vi "Begin.vi"(11 "Image Size":T1=enum."160x120") -> (0 "error out":errorcluster)   [LabVIEW 2012]
doc: "Called before other user functions, this VI is expected to open initial I/O refnums, load in file data, and do all program initialization. Notice that the <B>error out</B> terminal is simply used for data flow. Wiring it to other structures or subVIs ensures that this VI runs first."
uses:
  <vilib>/Rock Robotics/WPI/Camera/WPI_CameraImageSize.ctl
  <vilib>/Rock Robotics/WPI/Camera/WPI_CameraWhite Balance Values.ctl
  <vilib>/Rock Robotics/WPI/Camera/WPI_CameraExposure Values.ctl
  <vilib>/Rock Robotics/WPI/Camera/WPI_CameraFrameRate.ctl
  <vilib>/Rock Robotics/WPI/DriverStation/WPI_DriverStationRobotMode2.ctl
  <vilib>/Rock Robotics/WPI/Joystick/WPI_JoystickDeviceEnum.ctl
  <vilib>/Rock Robotics/SystemInterfaces/DIO/FPGA_DIOPWMChannel.ctl
  <vilib>/Rock Robotics/WPI/SafetyOutput/WPI_SafetyOutputConfigMenu.ctl
  <vilib>/Rock Robotics/SystemInterfaces/DIO/FPGA_DIORelayChannel.ctl
  <vilib>/Rock Robotics/SystemInterfaces/DIO/FPGA_DIOChannel.ctl
  <vilib>/Rock Robotics/WPI/Solenoid/WPI_SolenoidChannel.ctl
  <vilib>/Rock Robotics/SystemInterfaces/Typedef/FPGA_TypedefDigitalModule.ctl
  Robot Global Data.vi
  <vilib>/Rock Robotics/WPI/RobotDrive/WPI_RobotDriveOpen4MotorWithJaguar.vi
  <vilib>/Rock Robotics/WPI/MotorControl/WPI_MotorControlOpen Victor.vi
  <vilib>/Rock Robotics/WPI/Solenoid/WPI_SolenoidOpenSingle.vi
  <vilib>/Rock Robotics/WPI/Compressor/WPI_CompressorGetSetRefNum.vi
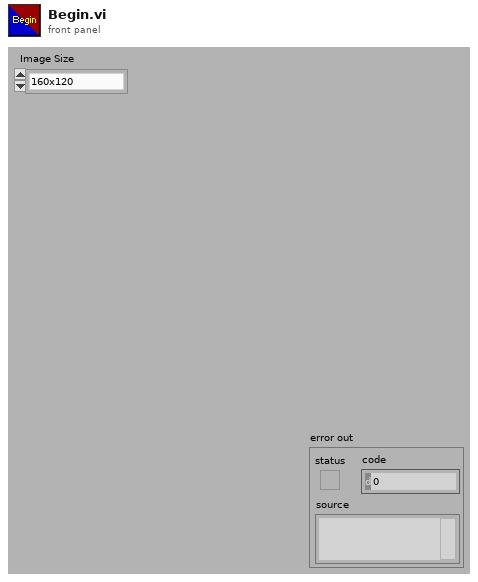
[diagram p1: front panel]
types:
  T1 = typedef "WPI_CameraImageSize.ctl" = enum16{"640x480", "320x240", "160x120"}
  T2 = typedef "FPGA_DIOPWMChannel.ctl" = enum8{"PWM 1", "PWM 2", "PWM 3", "PWM 4", "PWM 5", "PWM 6", "PWM 7", "PWM 8", "PWM 9", "PWM 10", "Invalid"}
  T3 = typedef "WPI_JoystickDeviceEnum.ctl" = enum16{"USB 1", "USB 2", "USB 3", "USB 4", "Kinect 1", "Kinect 2"}
  T4 = typedef "WPI_SafetyOutputConfigMenu.ctl" = enum16{"Enable", "Disable"}
  T5 = typedef "WPI_DriverStationRobotMode2.ctl" = enum16{"Autonomous Disabled", "Autonomous Enabled", "Teleop Disabled", "Teleop Enabled", "Timeout", "Finish", "Test Disabled", "Test Enabled"}
  T6 = typedef "WPI_CameraFrameRate.ctl" = u32
  T7 = typedef "WPI_CameraExposure Values.ctl" = enum16{"Auto", "Flicker-free 50 Hz", "Flicker-free 60 Hz", "Hold current"}
  T8 = typedef "WPI_CameraWhite Balance Values.ctl" = enum16{"Auto", "Fixed indoor", "Fixed outdoor 1", "Fixed outdoor 2", "Fixed fluorescent 1", "Fixed fluorescent 2", "Hold current"}
  T9 = typedef "WPI_SolenoidChannel.ctl" = enum8{"Solenoid 1", "Solenoid 2", "Solenoid 3", "Solenoid 4", "Solenoid 5", "Solenoid 6", "Solenoid 7", "Solenoid 8", "Invalid"}
  T10 = typedef "FPGA_DIOChannel.ctl" = enum8{"DIO 1", "DIO 2", "DIO 3", "DIO 4", "DIO 5", "DIO 6", "DIO 7", "DIO 8", "DIO 9", "DIO 10", "DIO 11", "DIO 12", "DIO 13", "DIO 14", "Invalid"}
  T11 = typedef "FPGA_DIORelayChannel.ctl" = enum8{"Relay 1", "Relay 2", "Relay 3", "Relay 4", "Relay 5", "Relay 6", "Relay 7", "Relay 8", "Invalid"}
  T12 = typedef "FPGA_TypedefDigitalModule.ctl" = enum16{"Digital Module 1", "Digital Module 2"}
  T13 = typedef "WPI_SolenoidDevRef.ctl" = cluster{"DevStatus":errorcluster, "Solenoid Module":T14, "Forward Solenoid Channel":T9, "Reverse Solenoid Channel":T9}
  T14 = typedef "FPGA_TypedefSolenoidModule.ctl" = enum16{"Solenoid Module 1", "Solenoid Module 2"}
  T15 = typedef "WPI_CompressorDevRef.ctl" = cluster{"DevStatus":errorcluster, "DigitalInputDevRef":T16, "RelayDevRef":T17}
  T16 = typedef "WPI_DigitalInputDevRef.ctl" = cluster{"DevStatus":errorcluster, "DIO Channel":T10, "Digital Module":T12}
  T17 = typedef "WPI_RelayDevRef.ctl" = cluster{"DevStatus":errorcluster, "Relay Channel":T11, "Digital Module":T12, "Relay Direction":T18}
  T18 = typedef "WPI_RelayDirection.ctl" = enum16{"Both directions", "Forward only", "Reverse only"}
  T19 = typedef "FPGA_WatchdogDevRef.ctl" = cluster{"DevStatus":errorcluster}
  T20 = typedef "WPI_RobotDriveDevRef.ctl" = cluster{"DevStatus":errorcluster, "Motors[]":T21[], "Square Inputs":bool, "Max Output":dbl, "Isochronous":bool}
  T21 = typedef "WPI_MotorControlDeviceRef.ctl" = cluster{"DeviceStatus":errorcluster, "Type":enum16{"PWM", "CAN"}, "PWM":cluster{"Digital Module":T12, "PWM Channel":T2, "DeadBand":T22}, "CAN":cluster{"Device Number":u8, "Control Mode":T23, "Semaphore":T24, "Max Vout":dbl}, "Invert":bool, "TransformRef":T25, "InvTransformRef":T25}
  T22 = typedef "WPI_PWMDeadband.ctl" = cluster{"Name":string, "maxPositivePwm":i32, "minPositivePwm":i32, "centerPwm":i32, "maxNegativePwm":i32, "minNegativePwm":i32, "angularRange":u16}
  T23 = typedef "WPI_CANJaguar_ControlMode.ctl" = enum8{"Percent VBus", "Current", "Speed", "Position", "Voltage"}
  T24 = typedef "Semaphore RefNum" = refnum<k1>
  T25 = typedef "WPI_PWMTransform_ConPane.ctl" = refnum<vi>
  T26 = typedef "WPI_JoystickDevRef.ctl" = cluster{"Device":T3}
  T27 = typedef "WPI_CameraDevRef.ctl" = cluster{"Camera Address":string, "CameraStatus":errorcluster, "Acquire Image Notifier":refnum<notifier>}
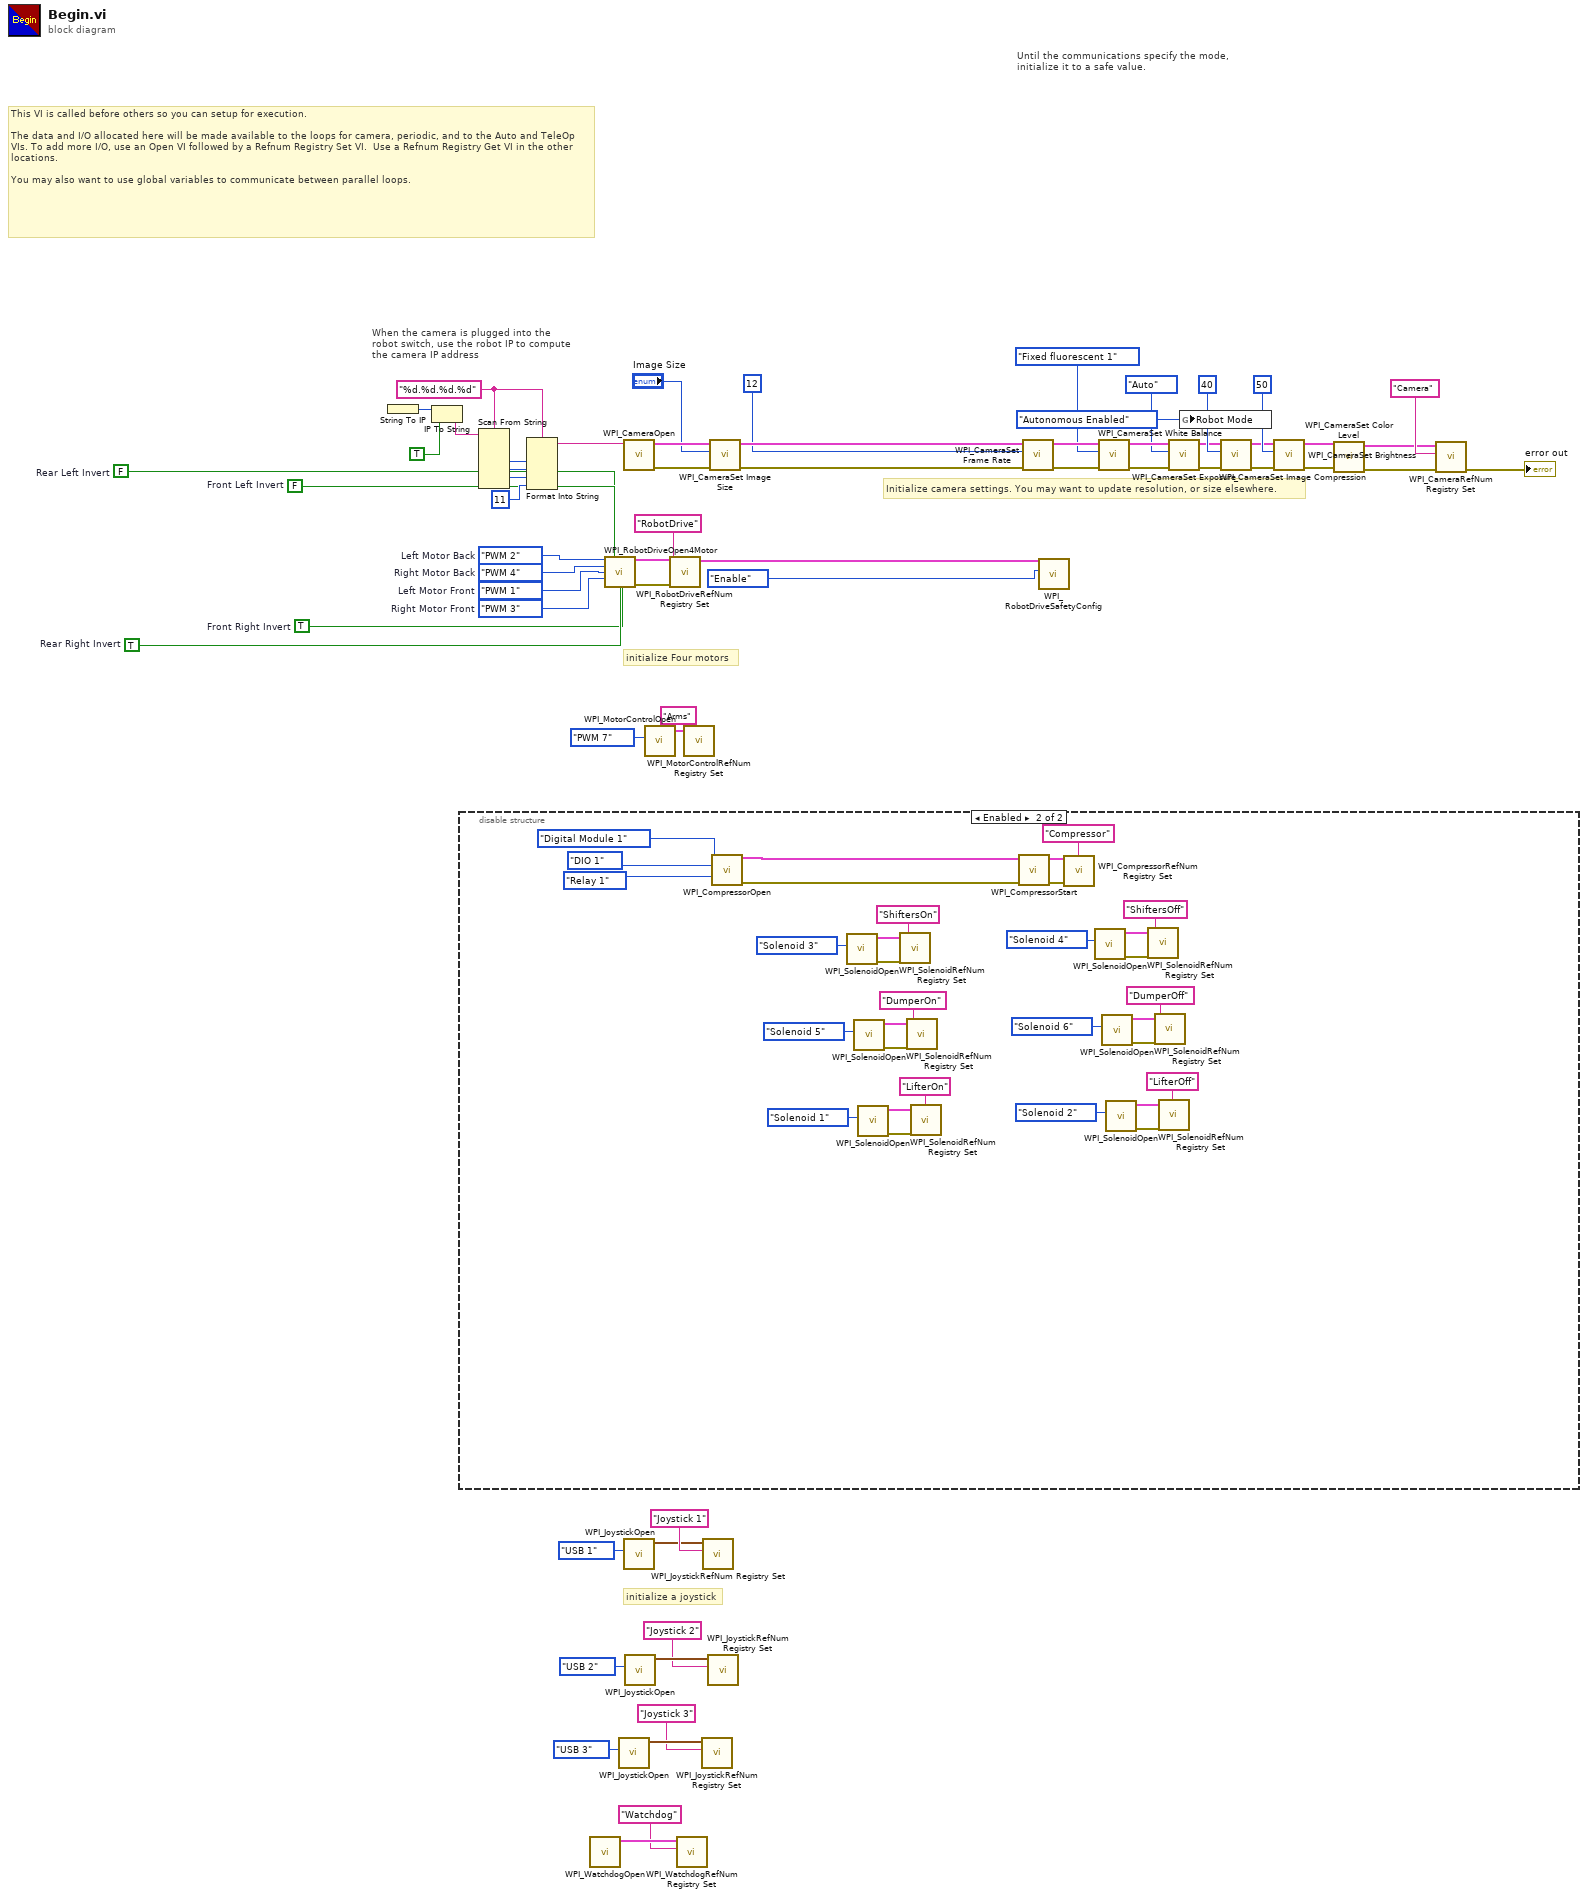
[diagram p0: block diagram]
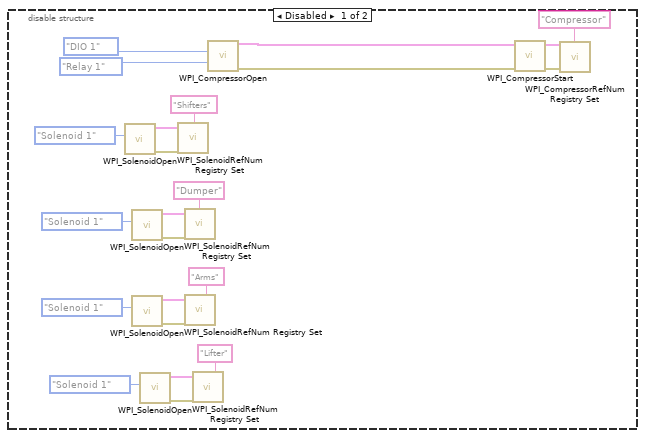
[diagram p2: hidden frame]
diagram:
  w16 = TRUE  # Front Right Invert
  w17 = FALSE  # Front Left Invert
  w22 = FPGA_DIOPWMChannel."PWM 4"  # Right Motor Back
  w19 = FPGA_DIOPWMChannel."PWM 3"  # Right Motor Front
  w21 = FPGA_DIOPWMChannel."PWM 2"  # Left Motor Back
  w20 = FPGA_DIOPWMChannel."PWM 1"  # Left Motor Front
  w15 = FALSE  # Rear Left Invert
  w18 = TRUE  # Rear Right Invert
  w35 = "%d.%d.%d.%d" ("format string")
  # "This VI is called before others so you can setup for execution.\n\nThe data and I/O allocated here will be made available to the loops for camera, periodic, and to the Auto and TeleOp VIs. To add more I/O, use an Open VI followed by a Refnum Registry Set VI.  Use a Refnum Registry Get VI in the other locations.\n\nYou may also want to use global variables to communicate between parallel loops."
  # "initialize a joystick"
  # "Until the communications specify the mode,\ninitialize it to a safe value."
  # "When the camera is plugged into the\nrobot switch, use the robot IP to compute\nthe camera IP address"
  # "initialize Four motors"
  # "Initialize camera settings. You may want to update resolution, or size elsewhere."
  n1 = String To IP() -> (0:w42:u32)  [unwired: 1 in]
  n2 = IP To String(1:TRUE ("dot notation? (F)"), 2:w42) -> (0:w40:string)
  n3 = disable-structure shown="Enabled" {
    frame Disabled {
      n4 = call-poly <vilib>:"WPI_SolenoidOpen.vi"("Solenoid Channel"=WPI_SolenoidChannel."Solenoid 1") -> ("error out"=w75:errorcluster, "SolenoidDevRef"=w76:T13)  [unwired: 9 in]
      n5 = call-poly <vilib>:"WPI_SolenoidOpen.vi"("Solenoid Channel"=WPI_SolenoidChannel."Solenoid 1") -> ("error out"=w71:errorcluster, "SolenoidDevRef"=w72:T13)  [unwired: 9 in]
      n6 = call-poly <vilib>:"WPI_SolenoidOpen.vi"("Solenoid Channel"=WPI_SolenoidChannel."Solenoid 1") -> ("error out"=w67:errorcluster, "SolenoidDevRef"=w68:T13)  [unwired: 9 in]
      n7 = call-poly <vilib>:"WPI_SolenoidOpen.vi"("Solenoid Channel"=WPI_SolenoidChannel."Solenoid 1") -> ("error out"=w63:errorcluster, "SolenoidDevRef"=w64:T13)  [unwired: 9 in]
      n8 = call <vilib>:"WPI_SolenoidRefNum Registry Set.vi"("error in (no error)"=w75, "refnum name"="Shifters", "SolenoidDevRef"=w76) -> ()  [unwired: 7 in, 2 out]
      n9 = call <vilib>:"WPI_SolenoidRefNum Registry Set.vi"("error in (no error)"=w71, "refnum name"="Dumper", "SolenoidDevRef"=w72) -> ()  [unwired: 7 in, 2 out]
      n10 = call <vilib>:"WPI_SolenoidRefNum Registry Set.vi"("error in (no error)"=w67, "refnum name"="Arms", "SolenoidDevRef"=w68) -> ()  [unwired: 7 in, 2 out]
      n11 = call <vilib>:"WPI_SolenoidRefNum Registry Set.vi"("error in (no error)"=w63, "refnum name"="Lifter", "SolenoidDevRef"=w64) -> ()  [unwired: 7 in, 2 out]
      n12 = call <vilib>:"WPI_CompressorOpen.vi"("Pressure Switch DIO Channel"=FPGA_DIOChannel."DIO 1", "Relay Channel"=FPGA_DIORelayChannel."Relay 1") -> ("CompressorDevRef"=w81:T15, "error out"=w82:errorcluster)  [unwired: 12 in]
      n13 = call <vilib>:"WPI_CompressorStart.vi"("error in (no error)"=w82, "CompressorDevRef"=w81) -> ("error out"=w79:errorcluster, "CompressorDevRef"=w80:T15)  [unwired: 8 in]
      n14 = call <vilib>:"WPI_CompressorRefNum Registry Set.vi"("error in (no error)"=w79, "refnum name"="Compressor", "CompressorDevRef"=w80) -> ()  [unwired: 7 in, 2 out]
    }
    frame Enabled {
      n15 = call <vilib>:"WPI_CompressorOpen.vi"("Pressure Switch Digital Module (Module 1)"=FPGA_TypedefDigitalModule."Digital Module 1", "Pressure Switch DIO Channel"=FPGA_DIOChannel."DIO 1", "Relay Channel"=FPGA_DIORelayChannel."Relay 1") -> ("CompressorDevRef"=w102:T15, "error out"=w101:errorcluster)  [unwired: 11 in]
      n16 = call-poly <vilib>:"WPI_SolenoidOpen.vi"("Solenoid Channel"=WPI_SolenoidChannel."Solenoid 3") -> ("error out"=w89:errorcluster, "SolenoidDevRef"=w88:T13)  [unwired: 9 in]
      n17 = call-poly <vilib>:"WPI_SolenoidOpen.vi"("Solenoid Channel"=WPI_SolenoidChannel."Solenoid 5") -> ("error out"=w93:errorcluster, "SolenoidDevRef"=w92:T13)  [unwired: 9 in]
      n18 = call-poly <vilib>:"WPI_SolenoidOpen.vi"("Solenoid Channel"=WPI_SolenoidChannel."Solenoid 1") -> ("error out"=w97:errorcluster, "SolenoidDevRef"=w96:T13)  [unwired: 9 in]
      n19 = call <vilib>:"WPI_SolenoidRefNum Registry Set.vi"("error in (no error)"=w89, "refnum name"="ShiftersOn", "SolenoidDevRef"=w88) -> ()  [unwired: 7 in, 2 out]
      n20 = call <vilib>:"WPI_SolenoidRefNum Registry Set.vi"("error in (no error)"=w93, "refnum name"="DumperOn", "SolenoidDevRef"=w92) -> ()  [unwired: 7 in, 2 out]
      n21 = call <vilib>:"WPI_SolenoidRefNum Registry Set.vi"("error in (no error)"=w97, "refnum name"="LifterOn", "SolenoidDevRef"=w96) -> ()  [unwired: 7 in, 2 out]
      n22 = call <vilib>:"WPI_CompressorStart.vi"("error in (no error)"=w101, "CompressorDevRef"=w102) -> ("error out"=w104:errorcluster, "CompressorDevRef"=w103:T15)  [unwired: 8 in]
      n23 = call <vilib>:"WPI_CompressorRefNum Registry Set.vi"("error in (no error)"=w104, "refnum name"="Compressor", "CompressorDevRef"=w103) -> ()  [unwired: 7 in, 2 out]
      n24 = call-poly <vilib>:"WPI_SolenoidOpen.vi"("Solenoid Channel"=WPI_SolenoidChannel."Solenoid 4") -> ("error out"=w108:errorcluster, "SolenoidDevRef"=w107:T13)  [unwired: 9 in]
      n25 = call-poly <vilib>:"WPI_SolenoidOpen.vi"("Solenoid Channel"=WPI_SolenoidChannel."Solenoid 6") -> ("error out"=w112:errorcluster, "SolenoidDevRef"=w111:T13)  [unwired: 9 in]
      n26 = call-poly <vilib>:"WPI_SolenoidOpen.vi"("Solenoid Channel"=WPI_SolenoidChannel."Solenoid 2") -> ("error out"=w116:errorcluster, "SolenoidDevRef"=w115:T13)  [unwired: 9 in]
      n27 = call <vilib>:"WPI_SolenoidRefNum Registry Set.vi"("error in (no error)"=w108, "refnum name"="ShiftersOff", "SolenoidDevRef"=w107) -> ()  [unwired: 7 in, 2 out]
      n28 = call <vilib>:"WPI_SolenoidRefNum Registry Set.vi"("error in (no error)"=w112, "refnum name"="DumperOff", "SolenoidDevRef"=w111) -> ()  [unwired: 7 in, 2 out]
      n29 = call <vilib>:"WPI_SolenoidRefNum Registry Set.vi"("error in (no error)"=w116, "refnum name"="LifterOff", "SolenoidDevRef"=w115) -> ()  [unwired: 7 in, 2 out]
    }
  }
  n30 = Scan From String(format string=w35, input string=w40) -> (output 1=w39:i32, output 2=w38:i32, output 3=w37:i32)  [unwired: 7 in, 3 out]
  n31 = Format Into String(format string=w35, w39, w38, w37, 11 ("Compression")) -> (resulting string=w34:string)  [unwired: 2 in, 1 out]
  n32 = call <vilib>:"WPI_WatchdogOpen.vi"() -> ("WatchdogDevRef"=w5:T19)  [unwired: 10 in, 1 out]
  n33 = call-poly <vilib>:"WPI_RobotDriveOpen4Motor.vi"("Rear Left Motor"=w21, "Rear Left Motor Inverted"=w15, "Rear Right Motor Inverted"=w18, "Rear Right Motor"=w22, "Front Left Motor"=w20, "Front Right Motor"=w19, "Front Left Motor Inverted"=w17, "Front Right Motor Inverted"=w16) -> ("RobotDriveDevRef"=w14:T20, "error out"=w13:errorcluster)  [unwired: 6 in]
  n34 = call <vilib>:"WPI_JoystickOpen.vi"("JoystickDevice"=WPI_JoystickDeviceEnum."USB 3") -> ("JoystickDevRef"=w7:T26)  [unwired: 10 in]
  n35 = call <vilib>:"WPI_CameraOpen.vi"("Camera Address"=w34) -> ("error out"=w52:errorcluster, "CameraDevRef"=w53:T27)  [unwired: 1 in, 8 out]
  n36 = call <vilib>:"WPI_JoystickOpen.vi"("JoystickDevice"=WPI_JoystickDeviceEnum."USB 1") -> ("JoystickDevRef"=w32:T26)  [unwired: 10 in]
  n37 = call <vilib>:"WPI_JoystickOpen.vi"("JoystickDevice"=WPI_JoystickDeviceEnum."USB 2") -> ("JoystickDevRef"=w28:T26)  [unwired: 10 in]
  n38 = call-poly <vilib>:"WPI_MotorControlOpen.vi"("PWM Channel"=FPGA_DIOPWMChannel."PWM 7") -> ("MotorControlDeviceRef"=w3:T21)  [unwired: 9 in, 1 out]
  n39 = call <vilib>:"WPI_RobotDriveRefNum Registry Set.vi"("error in (no error)"=w13, "refnum name"="RobotDrive", "RobotDriveDevRef"=w14) -> ("RobotDriveDevRef"=w11:T20)  [unwired: 8 out]
  n40 = call <vilib>:"WPI_WatchdogRefNum Registry Set.vi"("refnum name"="Watchdog", "WatchdogDevRef"=w5) -> ()  [unwired: 8 in, 2 out]
  n41 = call <vilib>:"WPI_MotorControlRefNum Registry Set.vi"("refnum name"="Arms", "MotorControlDevRef"=w3) -> ()  [unwired: 8 in, 2 out]
  n42 = call <vilib>:"WPI_JoystickRefNum Registry Set.vi"("refnum name"="Joystick 3", "JoystickDevRef"=w7) -> ()  [unwired: 8 in, 2 out]
  n43 = call <vilib>:"WPI_JoystickRefNum Registry Set.vi"("refnum name"="Joystick 1", "JoystickDevRef"=w32) -> ()  [unwired: 8 in, 2 out]
  n44 = call <vilib>:"WPI_JoystickRefNum Registry Set.vi"("refnum name"="Joystick 2", "JoystickDevRef"=w28) -> ()  [unwired: 8 in, 2 out]
  n45 = call <vilib>:"WPI_CameraSet Image Size.vi"("error in (no error)"=w52, "Image Size"="Image Size", "CameraDevRef"=w53) -> ("error out"=w51:errorcluster, "CameraDevRef Out"=w54:T27)  [unwired: 7 out]
  n46 = call <vilib>:"WPI_CameraSet Frame Rate.vi"("error in (no error)"=w51, "Frame Rate (fps)"=T6 12, "CameraDevRef"=w54) -> ("error out"=w50:errorcluster, "CameraDevRef Out"=w56:T27)  [unwired: 7 out]
  n47 = call <vilib>:"WPI_RobotDriveSafetyConfig.vi"("mode"=WPI_SafetyOutputConfigMenu."Enable", "RobotDriveDevRef"=w11) -> ()  [unwired: 8 in, 2 out]
  n48 = call <vilib>:"WPI_CameraSet White Balance.vi"("error in (no error)"=w50, "White Balance"=WPI_CameraWhite_Balance_Values."Fixed fluorescent 1", "CameraDevRef"=w56) -> ("error out"=w49:errorcluster, "CameraDevRef Out"=w55:T27)  [unwired: 7 out]
  n49 = call <vilib>:"WPI_CameraSet Exposure.vi"("error in (no error)"=w49, "Exposure"=WPI_CameraExposure_Values."Auto", "CameraDevRef"=w55) -> ("error out"=w48:errorcluster, "CameraDevRef Out"=w58:T27)  [unwired: 7 out]
  n50 = global write "Robot Global Data.vi" "Robot Mode"(WPI_DriverStationRobotMode2."Autonomous Enabled" ("Robot Mode")) -> ()
  n51 = call <vilib>:"WPI_CameraSet Image Compression.vi"("error in (no error)"=w48, "Compression"=40, "CameraDevRef"=w58) -> ("error out"=w47:errorcluster, "CameraDevRef Out"=w57:T27)  [unwired: 7 out]
  n52 = call <vilib>:"WPI_CameraSet Brightness.vi"("error in (no error)"=w47, "Brightness"=50, "CameraDevRef"=w57) -> ("error out"=w26:errorcluster, "CameraDevRef Out"=w25:T27)  [unwired: 7 out]
  n53 = call <vilib>:"WPI_CameraSet Color Level.vi"("error in (no error)"=w26, "CameraDevRef"=w25) -> ("error out"=w23:errorcluster, "CameraDevRef Out"=w24:T27)  [unwired: 8 in]
  n54 = call <vilib>:"WPI_CameraRefNum Registry Set.vi"("error in (no error)"=w23, "refnum name"="Camera", "CameraDevRef"=w24) -> ("error out"=→"error out":errorcluster)  [unwired: 8 out]
